vi "Select Target AO Channel.vi"(8 "error in (no error)":errorcluster, 10 "AO Channel":T2, 11 "Data in":T1) -> (0 "error out":errorcluster, 3 "Data out":T1)   [LabVIEW 2017, in "Test Bench.lvlib"]
uses:
  Test Bench.lvlib
  Scan Engine Variables.ctl
  <instrlib>/_niInstr/FIFO Register Bus/v1/Host/niInstr FIFO Register Bus v1 Host.lvclass
  <instrlib>/_niInstr/Instruction Framework/v1/Host/Instruction Framework Context/niInstr Instruction Framework Context v1 Host.lvclass
  AO Channels.ctl
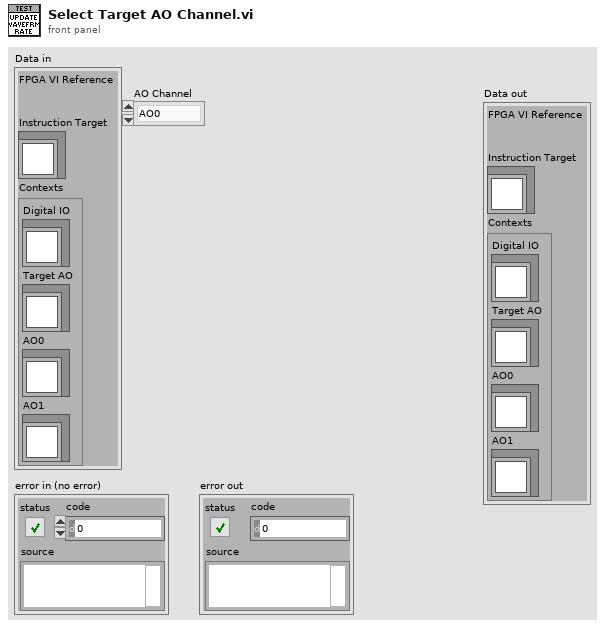
[diagram p1: front panel]
types:
  T1 = typedef "Test Bench.lvlib/Scan Engine Variables.ctl" = cluster{"FPGA VI Reference":refnum<k20>, "Instruction Target":refnum<class "niInstr FIFO Register Bus v1 Host.lvclass">, "Contexts":cluster{"Digital IO":refnum<class "niInstr Instruction Framework Context v1 Host.lvclass">, "Target AO":refnum<class "niInstr Instruction Framework Context v1 Host.lvclass">, "AO0":refnum<class "niInstr Instruction Framework Context v1 Host.lvclass">, "AO1":refnum<class "niInstr Instruction Framework Context v1 Host.lvclass">}}
  T2 = typedef "Test Bench.lvlib/AO Channels.ctl" = enum16{"AO0", "AO1"}
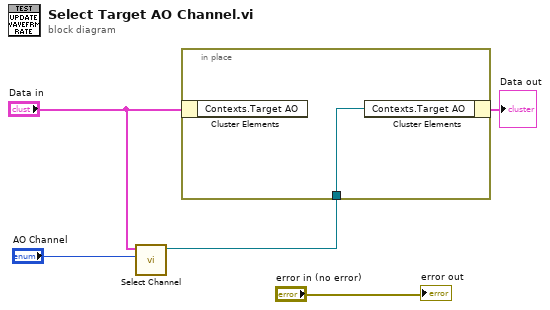
[diagram p0: block diagram]
diagram:
  n1 = call "Select Channel.vi"("AO Channel"="AO Channel", "Data"="Data in") -> ("Analog Output"=w2:refnum<class "niInstr Instruction Framework Context v1 Host.lvclass">)  [unwired: 9 in]
  n2 = in-place {
    in-place-border: w2 -> [w6]
    n3 = in-place-cluster #1("Data in") -> ()  [unwired: 1 out]
    n4 = in-place-cluster #1("Contexts.Target AO"=w6) -> (→"Data out":T1)
  }
  "error out" <- "error in (no error)"
